vi "Intersperse Data with Invalid Data 2parallel samples (multiple channel).vi"(1 "Intersperse Ratio":dbl=0.1, 5 "Channel0 Input":dbl[](array[numeric]) format="%.16g", 7 "Channel1 Input":dbl[](array[numeric]) format="%.16g") -> (6 "Channel0 Output":dbl[](array[numeric]), 8 "Channel1 Output":dbl[](array[numeric]), 10 "Data Valid":bool[](array[boolean]))   [LabVIEW 2011]
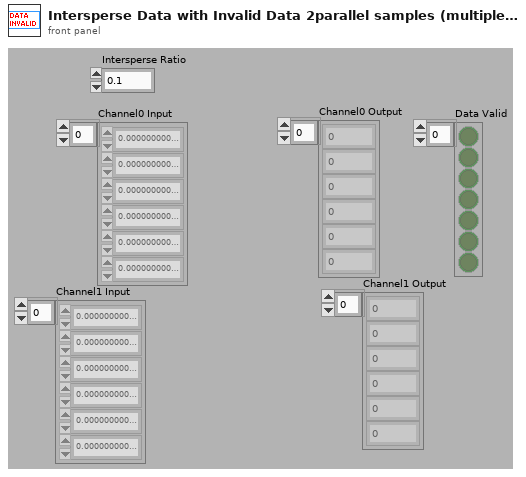
[diagram p1: front panel]
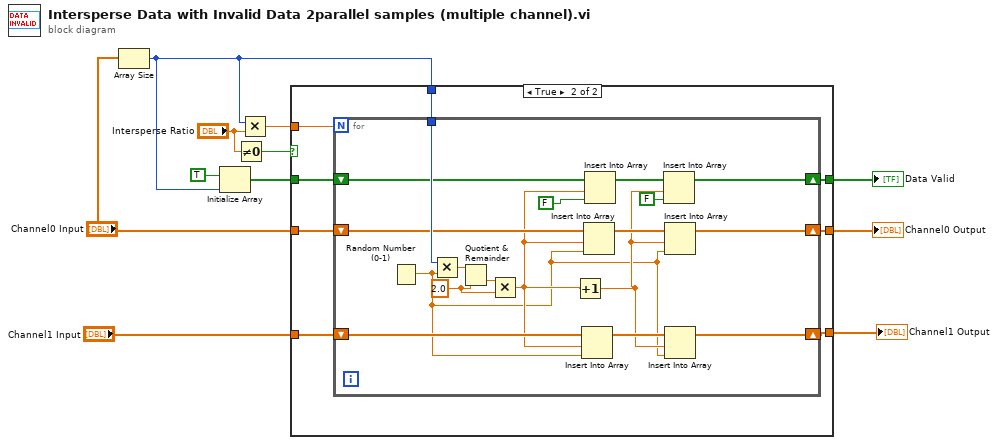
[diagram p0: block diagram]
diagram:
  n1 = Array Size(array="Channel0 Input") -> (size(s)=w10:i32)
  n2 = Initialize Array(TRUE, w10) -> (w8:bool[])
  n3 = Not Equal To 0?(x="Intersperse Ratio") -> (x != 0?=w1:bool)
  n4 = Multiply(x=w10, y="Intersperse Ratio") -> (x*y=w3:dbl)
  n5 = case shown="True" w1 {
    tunnel: "Channel0 Input" -> [w14 w22]
    tunnel: w10 -> [_ w21]
    tunnel: w8 -> [w13 w20]
    tunnel: [w13 w19] -> w7
    tunnel: [w14 w18] -> w6
    tunnel: "Channel1 Input" -> [w12 w17]
    tunnel: [w12 w16] -> w4
    tunnel: w3 -> [_ w15]
    frame False {
    }
    frame True {
      n6 = for {
        N: w15 -> [_]
        tunnel: w21 -> [w40]
        shift-right: [w29] -> w18
        shift-left: w22 -> [w39]
        shift-right: [w31] -> w19
        shift-left: w20 -> [w38]
        shift-right: [w27] -> w16
        shift-left: w17 -> [w37]
        w33 = 2.0 ("y")
        n7 = Random Number (0-1)() -> (number: 0 to 1=w23:dbl)
        n8 = Multiply(x=w40, y=w23) -> (x*y=w35:dbl)
        n9 = Quotient & Remainder(x=w35, y=w33) -> (floor(x/y)=w34:dbl)  [unwired: 1 out]
        n10 = Multiply(x=w34, y=w33) -> (x*y=w26:dbl)
        n11 = Increment(x=w26) -> (x+1=w25:dbl)
        n12 = Insert Into Array(array=w37, index=w26, new element=w23) -> (w28:dbl[])
        n13 = Insert Into Array(array=w39, index=w26, new element=w23) -> (w30:dbl[])
        n14 = Insert Into Array(array=w38, index=w26, new element=FALSE) -> (w32:bool[])
        n15 = Insert Into Array(array=w32, index=w25, new element=FALSE ("new element/subarray")) -> (w31:bool[])
        n16 = Insert Into Array(array=w30, index=w25, new element=w23) -> (w29:dbl[])
        n17 = Insert Into Array(array=w28, index=w25, new element=w23) -> (w27:dbl[])
      }
    }
  }
  "Data Valid" <- w7
  "Channel0 Output" <- w6
  "Channel1 Output" <- w4
